vi "泵温度校准配置.vi"() -> ()   [LabVIEW 2016, in "斯坦道CODMn新电路板.lvlib"]
uses:
  <vilib>/Utility/miscctls.llb/LVPointTypeDef.ctl
panel:
  in  "关闭":bool
  in  "偏心轮校准簇":T1={"复位"=FALSE, "进纯水"=FALSE, "停止"=FALSE, "液体重量"=60, "偏心轮校准"=FALSE}
  in  "温度校准簇":T2={"进纯水"=FALSE, "排液"=FALSE, "停止 2"=FALSE, "开始加热"=FALSE, "温度值"=115.0, "温度校准"=FALSE}
  # "偏心轮、温度校准"
  # "输入实际液体重量:"
  # "g"
  # "温度:"
  # "℃"
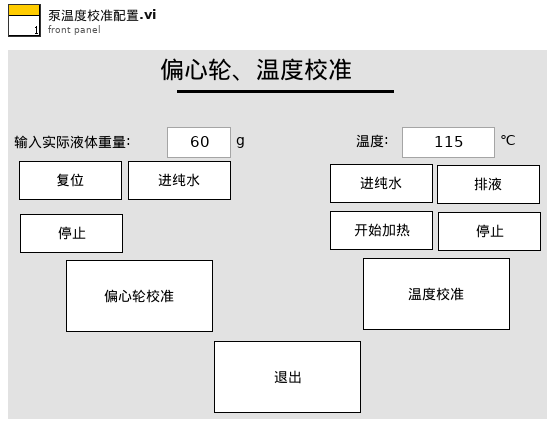
[diagram p1: front panel]
types:
  T1 = cluster{"复位":bool, "进纯水":bool, "停止":bool, "液体重量":u16, "偏心轮校准":bool}
  T2 = cluster{"进纯水":bool, "排液":bool, "停止 2":bool, "开始加热":bool, "温度值":dbl, "温度校准":bool}
  T3 = typedef "LVPointTypeDef.ctl" = cluster{"Horizontal":i16, "Vertical":i16}
  T4 = cluster{"泵类型":u8, "阀数量":u8, "纯水通道":u8, "废液通道":u8, "进样速度":u16, "出样速度":u16, "滴定速度":u16, "注射泵保温温度L":u8, "注射泵保温温度H":u8, "注射泵加热超时时间":u16, "是否存在液位检测板":u16, "A值告警下限值":u16, "A值告警上限值":u16, "B值告警下限值":u16, "B值告警上限值":u16, "AB跨度告警值":u16, "阀配置:":u8, "滴定等待时间":u16, "滴定吸光度斜率":dbl}
  T5 = cluster{"系统时间":timestamp, "工作状态":u16, "测量模式":enum16{"待机", "连续模式", "周期模式", "定点模式", "受控模式", "手动模式"}, "告警代码":u16, "故障代码":u16, "日志代码":u16, "软件版本":u16, "A":sgl, "B":sgl, "K":sgl, "当前滴定数":sgl, "T":sgl, "H":sgl, "id":u16, "flowid":u16, "量程":u16, "加热实时温度":sgl, "当前ORP值":sgl, "运行时间":sgl, "当前步骤剩余时间":sgl, "结束滴定数":sgl, "注射泵保温温度":sgl, "匹配滴定数X0":u16, "X^2":sgl, "X":sgl, "B 2":sgl, "光值1":sgl, "光值2":sgl, "光值3":sgl, "光值4":sgl, "光值5":sgl, "光值6":sgl, "光值7":sgl, "光值8":sgl}
  T6 = cluster{"偏心轮校准参数":dbl, "运行速度(修改需要重启)":u16, "加热温度(校准参数) ":dbl, "告警温度":dbl, "加热超时时间:(单位/秒)":dbl, "K p":dbl, "K i":dbl, "K d":dbl, "ILimitUp":dbl, "ILimitDown":dbl}
  T7 = cluster{"检出限":dbl, "测量精度":dbl, "上限":dbl, "下限":dbl, "阈值（低->高）":dbl, "阈值（高->低）":dbl}
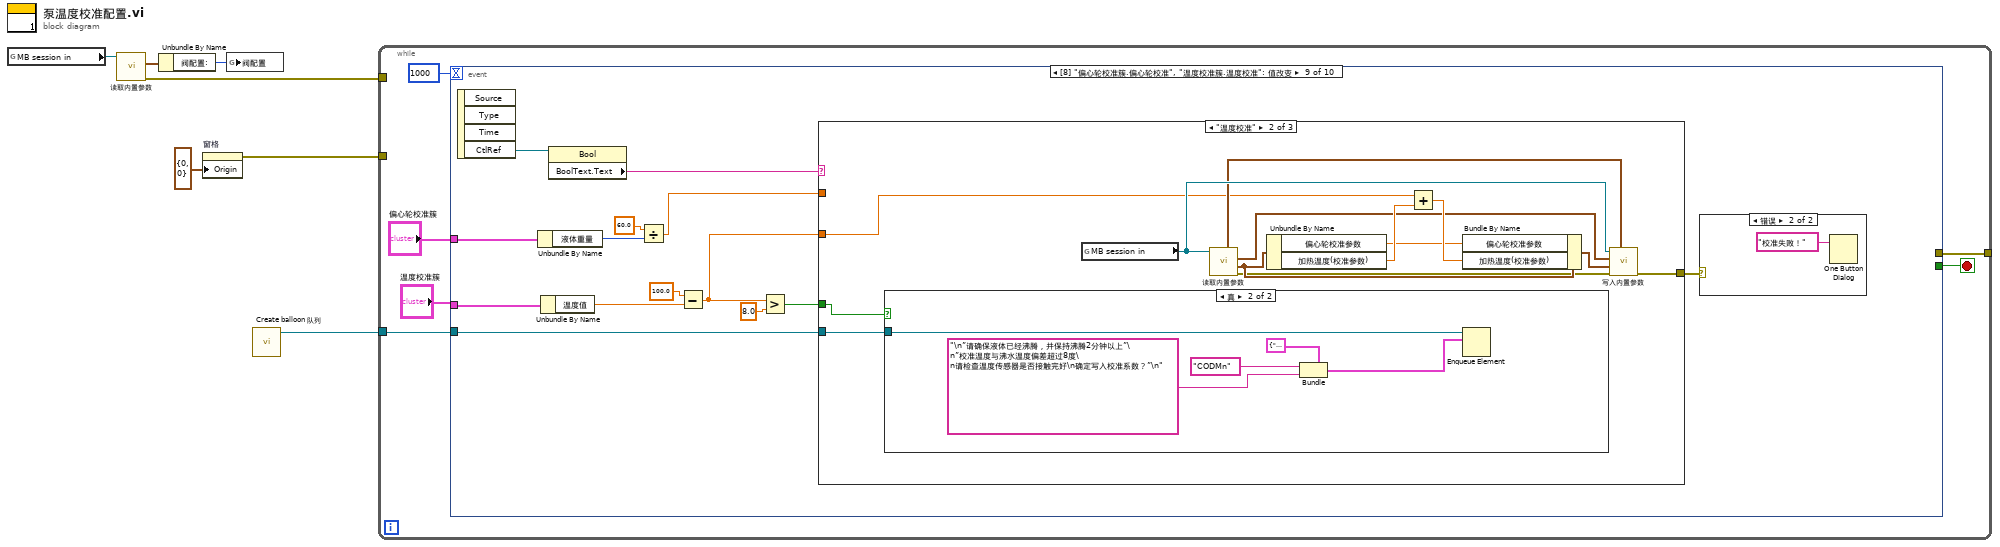
[diagram p0: block diagram]
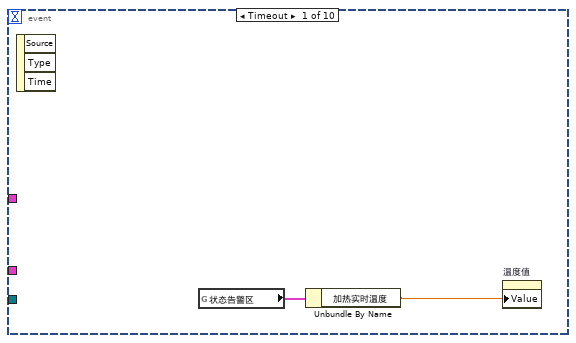
[diagram p2: hidden frame]
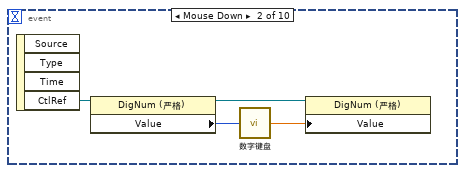
[diagram p3: hidden frame]
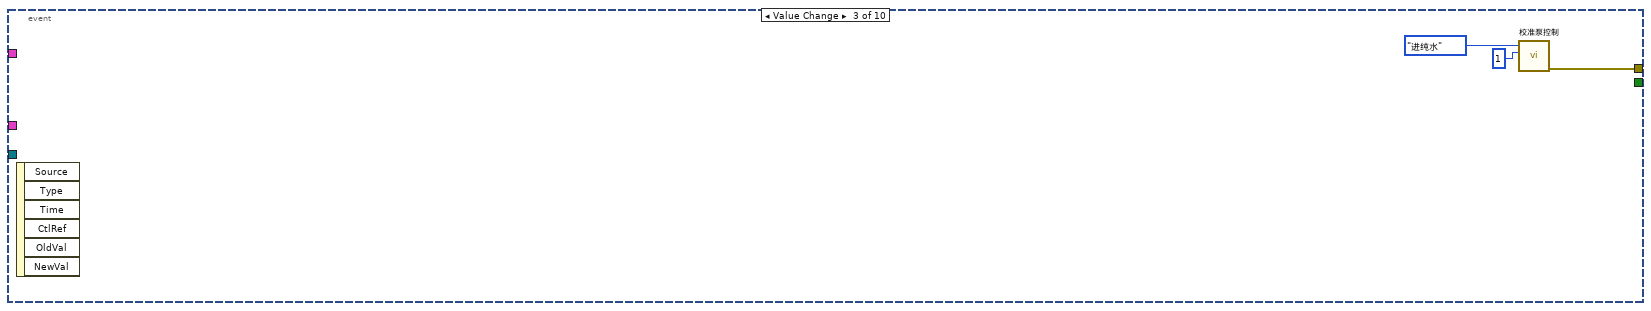
[diagram p4: hidden frame]
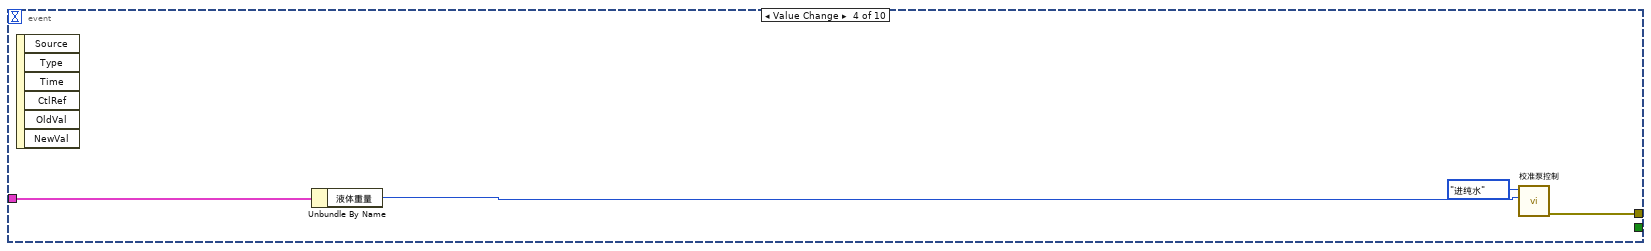
[diagram p5: hidden frame]
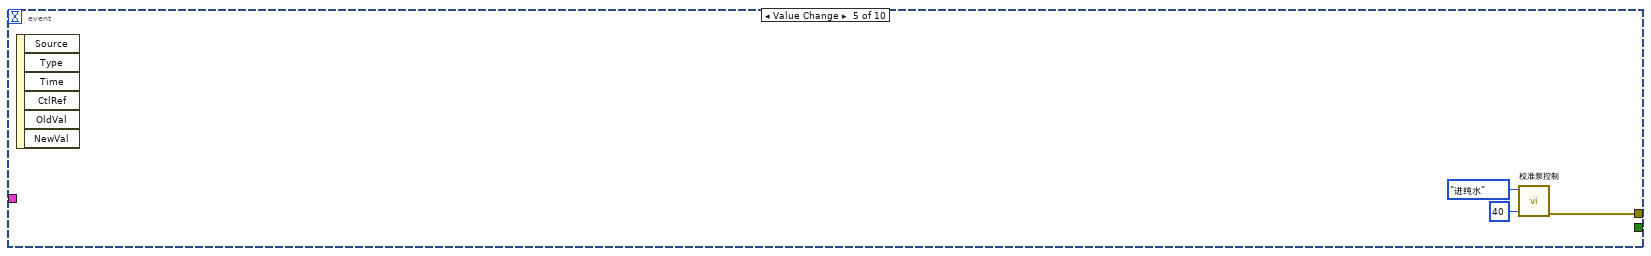
[diagram p6: hidden frame]
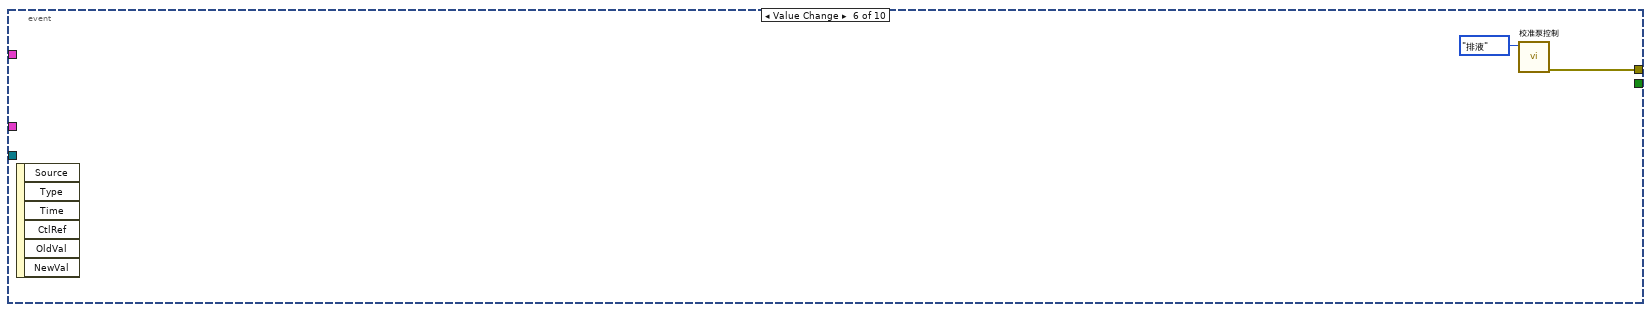
[diagram p7: hidden frame]
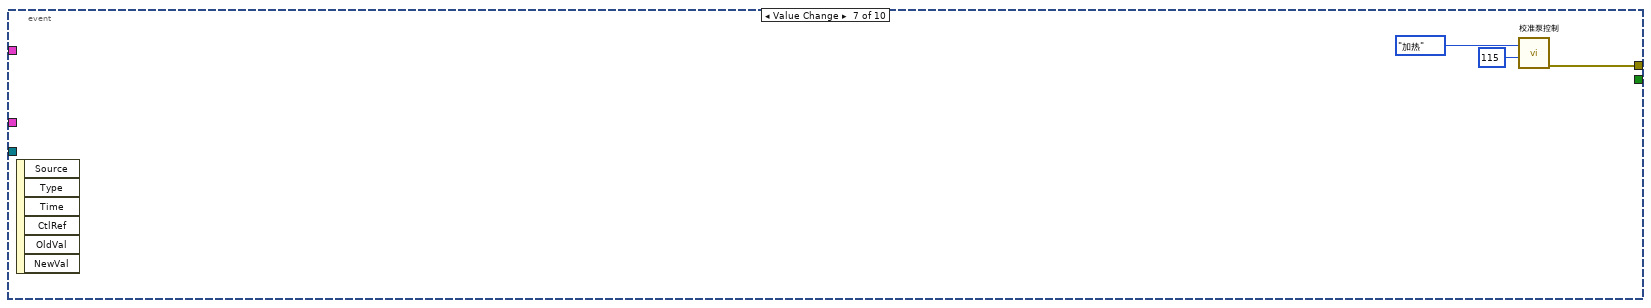
[diagram p8: hidden frame]
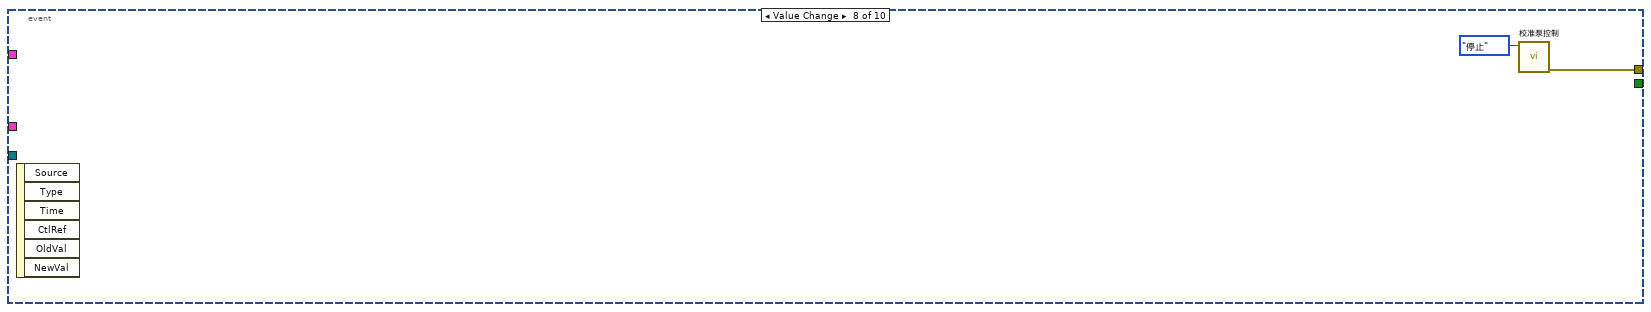
[diagram p9: hidden frame]
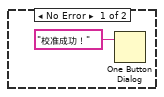
[diagram p10: hidden frame]
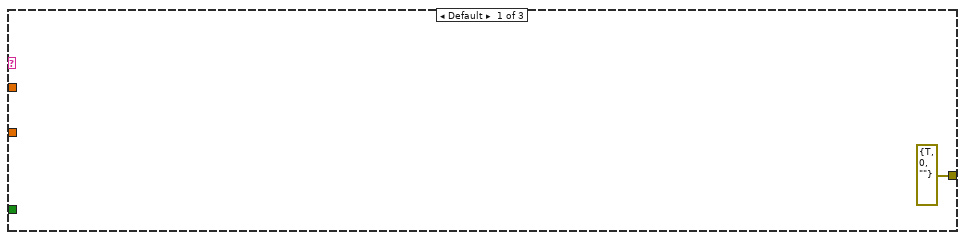
[diagram p11: hidden frame]
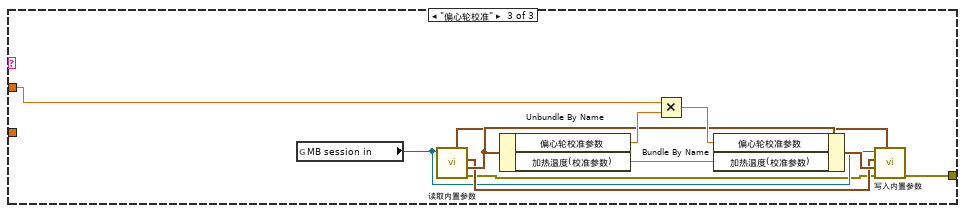
[diagram p13: hidden frame]
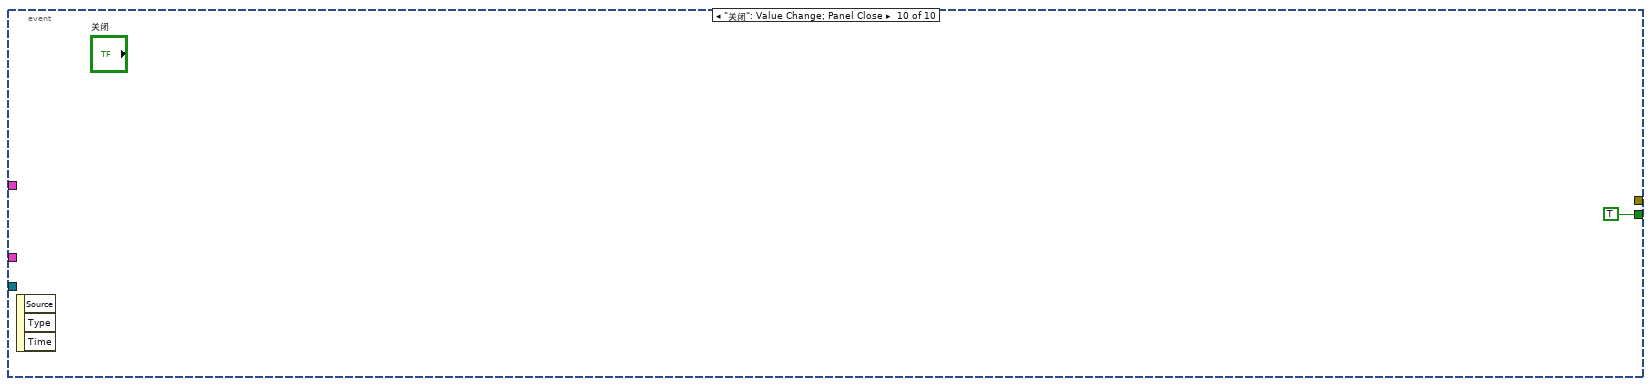
[diagram p14: hidden frame]
diagram:
  n1 = global read "VARCODMn全局变量.vi" "MB session in"() -> (w4:refnum<class "MB_Master.lvclass">)
  n2 = call "读取内置参数.vi"("MB session in"=w4) -> ("error out"=w1:errorcluster, "外设配置"=w3:T4)  [unwired: 6 in, 3 out]
  n3 = Unbundle By Name(w3) -> ("阀配置:"=w2:u8)
  n4 = property on="窗格" class="Pane"("Origin"=T3 {"Horizontal"=0, "Vertical"=0} ("原点")) -> (error out=w7:errorcluster)  [unwired: 2 in, 1 out]
  n5 = global write "CODMn断电保存全局变量.vi" "阀配置"(w2) -> ()
  n6 = call "Create balloon 队列.vi"() -> ("队列输出"=w5:refnum<queue>)  [unwired: 11 in]
  n7 = while {
    tunnel: w7 -> [_]
    tunnel: [w12] -> _
    tunnel: w5 -> [w10]
    tunnel: w1 -> [_]
    stop <- w13 stop-if-true
    n8 = event shown="[8] \"偏心轮校准簇.偏心轮校准\", \"温度校准簇.温度校准\": 值改变" {
      selector: _ -> [_ _ _ _ _ _ _ _ _ _]
      dyn-events: _ -> [_ _ _ _ _ _ _ _ _ _]
      timeout: 1000 -> [_ _ _ _ _ _ _ _ _ _]
      tunnel: [_ _ _ _ _ _ _ _ _ TRUE] -> w13
      tunnel: "偏心轮校准簇" -> [_ _ _ w25 _ _ _ _ w50 _]
      tunnel: [_ _ w21 w26 w29 w31 w34 w36 _ _] -> w12
      tunnel: "温度校准簇" -> [_ _ _ _ _ _ _ _ w37 _]
      tunnel: w10 -> [_ _ _ _ _ _ _ _ w39 _]
      event Timeout {
        n9 = event-data() -> ()  [unwired: 1 in, 3 out]
        n10 = global read "VARCODMn全局变量.vi" "状态告警区"() -> (w15:T5)
        n11 = Unbundle By Name(w15) -> ("加热实时温度"=w14:sgl)
        n12 = property on="温度值" class="DigNum (严格)"("Value"=w14) -> ()  [unwired: 2 in, 2 out]
      }
      event "偏心轮校准簇.液体重量": Mouse Down {
        n13 = event-data() -> ("CtlRef"=w16:refnum<vi>)  [unwired: 1 in, 3 out]
        n14 = property class="DigNum (严格)"(reference=w16) -> (reference out=w18:refnum<vi>, "Value"=w19:u16)  [unwired: 1 in, 1 out]
        n15 = call "数字键盘.vi"("OldNumber"=w19) -> ("NewNumber"=w17:dbl)
        n16 = property class="DigNum (严格)"(reference=w18, "Value"=w17) -> ()  [unwired: 1 in, 2 out]
      }
      event "偏心轮校准簇.复位": Value Change {
        n17 = event-data() -> ()  [unwired: 1 in, 6 out]
        n18 = call "校准泵控制.vi"("偏心轮"=u16 1, "枚举"=enum16{"进水样", "进纯水", "排液", "加热", "停止"}."进纯水") -> ("错误输出"=w21:errorcluster)  [unwired: 9 in]
      }
      event "偏心轮校准簇.进纯水": Value Change {
        n19 = event-data() -> ()  [unwired: 1 in, 6 out]
        n20 = Unbundle By Name(w25) -> ("液体重量"=w24:u16)
        n21 = call "校准泵控制.vi"("偏心轮"=w24, "枚举"=enum16{"进水样", "进纯水", "排液", "加热", "停止"}."进纯水") -> ("错误输出"=w26:errorcluster)  [unwired: 9 in]
      }
      event "温度校准簇.进纯水": Value Change {
        n22 = event-data() -> ()  [unwired: 1 in, 6 out]
        n23 = call "校准泵控制.vi"("偏心轮"=u16 40, "枚举"=enum16{"进水样", "进纯水", "排液", "加热", "停止"}."进纯水") -> ("错误输出"=w29:errorcluster)  [unwired: 9 in]
      }
      event "温度校准簇.排液": Value Change {
        n24 = event-data() -> ()  [unwired: 1 in, 6 out]
        n25 = call "校准泵控制.vi"("枚举"=enum16{"进水样", "进纯水", "排液", "加热", "停止"}."排液") -> ("错误输出"=w31:errorcluster)  [unwired: 10 in]
      }
      event "温度校准簇.开始加热": Value Change {
        n26 = event-data() -> ()  [unwired: 1 in, 6 out]
        n27 = call "校准泵控制.vi"("摄氏度"=u16 115, "枚举"=enum16{"进水样", "进纯水", "排液", "加热", "停止"}."加热") -> ("错误输出"=w34:errorcluster)  [unwired: 9 in]
      }
      event "温度校准簇.停止 2", "偏心轮校准簇.停止": Value Change {
        n28 = event-data() -> ()  [unwired: 1 in, 6 out]
        n29 = call "校准泵控制.vi"("枚举"=enum16{"进水样", "进纯水", "排液", "加热", "停止"}."停止") -> ("错误输出"=w36:errorcluster)  [unwired: 10 in]
      }
      event "偏心轮校准簇.偏心轮校准", "温度校准簇.温度校准": Value Change {
        n30 = event-data() -> ("CtlRef"=w44:refnum<vi>)  [unwired: 1 in, 3 out]
        n31 = Unbundle By Name(w50) -> ("液体重量"=w48:u16)
        n32 = Unbundle By Name(w37) -> ("温度值"=w46:dbl)
        n33 = property class="Bool"(reference=w44) -> ("BoolText.Text"=w41:string)  [unwired: 1 in, 2 out]
        n34 = Divide(x=60.0, y=w48) -> (x/y=w43:dbl)
        n35 = Subtract(x=100.0, y=w46) -> (x-y=w42:dbl)
        n36 = Greater?(x=w42, y=8.0) -> (0:w40:bool)
        n37 = case shown="\"温度校准\"" w41 {
          tunnel: w43 -> [_ _ w74]
          tunnel: w42 -> [_ w56 _]
          tunnel: w40 -> [_ w58 _]
          tunnel: w39 -> [_ w57 _]
          tunnel: [errorcluster {"status"=TRUE, "code"=0, "source"=""} ("error out") w54 w72] -> w38
          frame Default {
          }
          frame "温度校准" {
            n38 = case shown="真" w58 {
              tunnel: w57 -> [_ w71]
              frame False {
              }
              frame True {
                n39 = Bundle(cluster=cluster{"Title":string, "Body":string} {"Title"="", "Body"=""} ("元素"), "Title"="CODMn", "Body"="\n”请确保液体已经沸腾，并保持沸腾2分钟以上”\n”校准温度与沸水温度偏差超过8度\n请检查温度传感器是否接触完好\n确定写入校准系数？”\n") -> (w67:cluster{"Title":string, "Body":string})
                n40 = Enqueue Element(queue=w71, element=w67) -> ()  [unwired: 2 in, 3 out]
              }
            }
            n41 = global read "VARCODMn全局变量.vi" "MB session in"() -> (w61:refnum<class "MB_Master.lvclass">)
            n42 = call "读取内置参数.vi"("MB session in"=w61) -> ("error out"=w59:errorcluster, "float"=w63:T6, "外设配置"=w62:T4, "量程参数读取"=w60:T7)  [unwired: 6 in, 1 out]
            n43 = Unbundle By Name(w63) -> ("偏心轮校准参数"=w55:dbl, "加热温度(校准参数)"=w65:dbl)
            n44 = Add(x=w56, y=w65) -> (x+y=w66:dbl)
            n45 = Bundle By Name(cluster=w63, "偏心轮校准参数"=w55, "加热温度(校准参数)"=w66) -> (w64:T6)
            n46 = call "写入内置参数.vi"("量程参数读取"=w60, "error in (no error)"=w59, "float"=w64, "外设配置"=w62, "MB session in"=w61) -> ("error out"=w54:errorcluster)  [unwired: 5 in, 1 out]
          }
          frame "偏心轮校准" {
            n47 = global read "VARCODMn全局变量.vi" "MB session in"() -> (w77:refnum<class "MB_Master.lvclass">)
            n48 = call "读取内置参数.vi"("MB session in"=w77) -> ("error out"=w75:errorcluster, "float"=w79:T6, "外设配置"=w78:T4, "量程参数读取"=w76:T7)  [unwired: 6 in, 1 out]
            n49 = Unbundle By Name(w79) -> ("偏心轮校准参数"=w81:dbl, "加热温度(校准参数)"=w73:dbl)
            n50 = Multiply(x=w74, y=w81) -> (x*y=w82:dbl)
            n51 = Bundle By Name(cluster=w79, "偏心轮校准参数"=w82, "加热温度(校准参数)"=w73) -> (w80:T6)
            n52 = call "写入内置参数.vi"("量程参数读取"=w76, "error in (no error)"=w75, "float"=w80, "外设配置"=w78, "MB session in"=w77) -> ("error out"=w72:errorcluster)  [unwired: 5 in, 1 out]
          }
        }
        n53 = case shown="错误" w38 {
          frame No Error {
            n54 = One Button Dialog(message="校准成功！" ("消息")) -> ()  [unwired: 1 in, 1 out]
          }
          frame Error {
            n55 = One Button Dialog(message="校准失败！" ("消息")) -> ()  [unwired: 1 in, 1 out]
          }
        }
      }
      event "关闭": Value Change; Panel Close {
        n56 = event-data() -> ()  [unwired: 1 in, 3 out]
      }
    }
  }
